vi "Deadband Mecanum.vi"(3 "Axes 2 and 3 Deadband Input":dbl, 4 "Axes 1 Deadband Input":dbl, 5 "Axes 4 Deadband Input":dbl) -> (0 "Axes 2 and 3 Deadband Output":dbl, 1 "Axes 1 Deadband Output":dbl, 2 "Axes 4 Deadband Output":dbl)   [LabVIEW 2015]
panel:
  # "Axes 2 and 3 should be connected together because the \nare linked to the rotation of the mecanum drive."
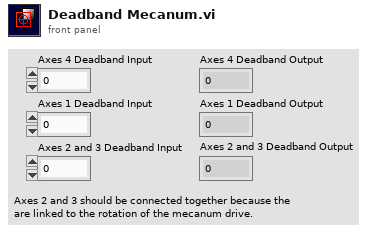
[diagram p1: front panel]
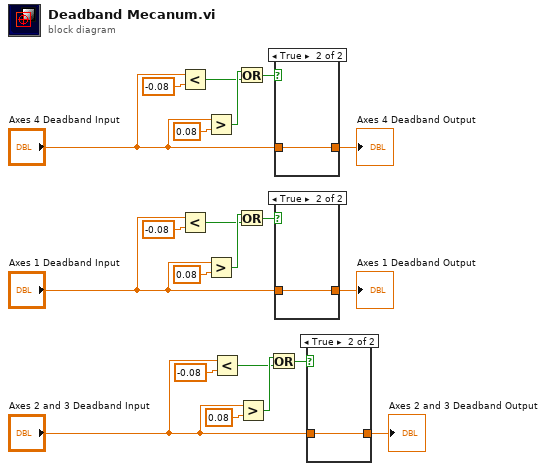
[diagram p0: block diagram]
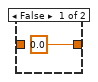
[diagram p2: hidden frame]
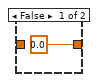
[diagram p3: hidden frame]
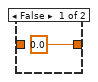
[diagram p4: hidden frame]
diagram:
  n1 = Less?(x="Axes 4 Deadband Input", y=-0.08) -> (x < y?=w19:bool)
  n2 = Less?(x="Axes 1 Deadband Input", y=-0.08) -> (x < y?=w13:bool)
  n3 = Greater?(x="Axes 4 Deadband Input", y=0.08) -> (0:w20:bool)
  n4 = Greater?(x="Axes 1 Deadband Input", y=0.08) -> (0:w14:bool)
  n5 = Less?(x="Axes 2 and 3 Deadband Input", y=-0.08) -> (x < y?=w8:bool)
  n6 = Or(x=w20, y=w19) -> (x .or. y?=w18:bool)
  n7 = Or(x=w14, y=w13) -> (x .or. y?=w12:bool)
  n8 = Greater?(x="Axes 2 and 3 Deadband Input", y=0.08) -> (0:w9:bool)
  n9 = Or(x=w9, y=w8) -> (x .or. y?=w7:bool)
  n10 = case shown="True" w18 {
    tunnel: [0.0 ("Joystick Arcband Input") w23] -> w21
    tunnel: "Axes 4 Deadband Input" -> [_ w23]
    frame False {
    }
    frame True {
    }
  }
  "Axes 4 Deadband Output" <- w21
  n11 = case shown="True" w12 {
    tunnel: [0.0 ("Joystick Arcband Input") w25] -> w2
    tunnel: "Axes 1 Deadband Input" -> [_ w25]
    frame False {
    }
    frame True {
    }
  }
  "Axes 1 Deadband Output" <- w2
  n12 = case shown="True" w7 {
    tunnel: [0.0 ("Joystick Arcband Input") w27] -> w1
    tunnel: "Axes 2 and 3 Deadband Input" -> [_ w27]
    frame False {
    }
    frame True {
    }
  }
  "Axes 2 and 3 Deadband Output" <- w1
